vi "ZAD_5_PART_1.vi"() -> ()   [LabVIEW 2023]
panel:
  out "Array":bool[](array[boolean])
  in  "Boolean 8":bool=TRUE
  in  "stop":bool
  in  "Enum":enum16{"XOR", "OR", "AND"}(ring)
  out "Boolean 24":bool
  out "Boolean 23":bool
  out "Boolean 22":bool
  out "Boolean 21":bool
  out "Boolean 20":bool
  out "Boolean 19":bool
  out "Boolean 18":bool
  out "Boolean 17":bool
  in  "Boolean 16":bool
  in  "Boolean 15":bool
  in  "Boolean 14":bool
  in  "Boolean 13":bool
  in  "Boolean 12":bool
  in  "Boolean 11":bool
  in  "Boolean 10":bool
  in  "Boolean 9":bool
  in  "Boolean 7":bool
  in  "Boolean 6":bool
  in  "Boolean 5":bool
  in  "Boolean 4":bool
  in  "Boolean 3":bool
  in  "Boolean 2":bool
  in  "Boolean":bool
  # "Bajt 1"
  # "Bajt 2"
  # "Wynik"
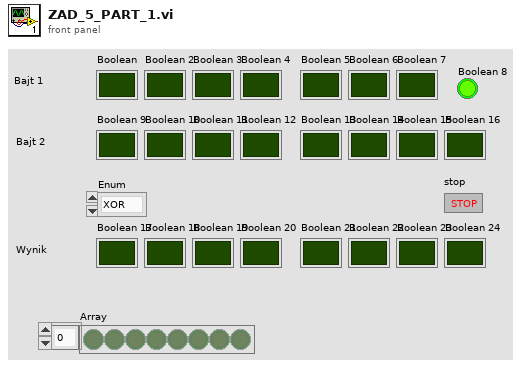
[diagram p1: front panel]
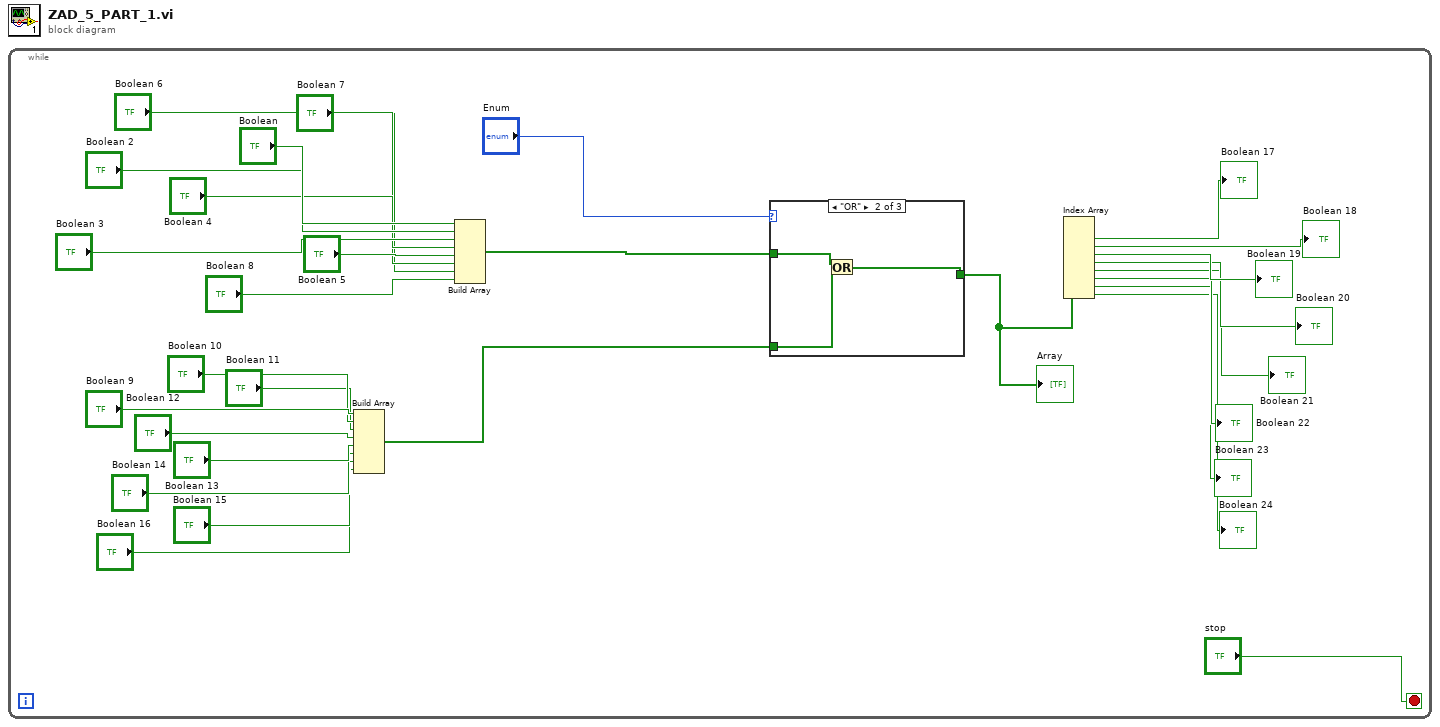
[diagram p0: block diagram]
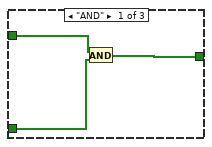
[diagram p2: hidden frame]
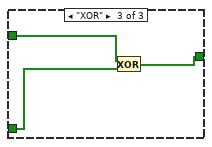
[diagram p3: hidden frame]
diagram:
  n1 = while {
    stop <- "stop" stop-if-true
    n2 = Build Array("Boolean 9", "Boolean 10", "Boolean 11", "Boolean 12", "Boolean 13", "Boolean 14", "Boolean 15", "Boolean 16") -> (w12:bool[])
    n3 = Build Array("Boolean", "Boolean 2", "Boolean 3", "Boolean 4", "Boolean 5", "Boolean 6", "Boolean 7", "Boolean 8") -> (w11:bool[])
    n4 = case shown="\"OR\"" "Enum" {
      tunnel: w12 -> [w31 w34 w37]
      tunnel: w11 -> [w32 w35 w38]
      tunnel: [w30 w33 w36] -> w10
      frame "AND" {
        n5 = And(x=w32, y=w31) -> (x .and. y?=w30:bool[])
      }
      frame "OR" {
        n6 = Or(x=w35, y=w34) -> (x .or. y?=w33:bool[])
      }
      frame "XOR" {
        n7 = Exclusive Or(1:w37, 2:w38) -> (0:w36:bool[])
      }
    }
    "Array" <- w10
    n8 = Index Array(array=w10) -> (element #1=→"Boolean 17":bool, element #2=→"Boolean 18":bool, element #3=→"Boolean 19":bool, element #4=→"Boolean 20":bool, element #5=→"Boolean 21":bool, element #6=→"Boolean 22":bool, element #7=→"Boolean 23":bool, element #8=→"Boolean 24":bool)  [unwired: 8 in]
  }
